vi "changeFWpos.vi"(1 "FW pos":u8, 2 "FWhandle":u32) -> (0 "fwPosChanged":bool)   [LabVIEW 2015]
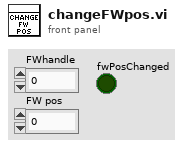
[diagram p1: front panel]
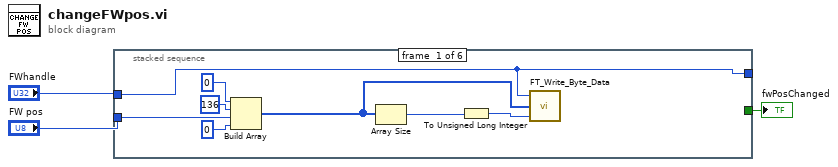
[diagram p0: block diagram]
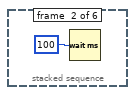
[diagram p2: hidden frame]
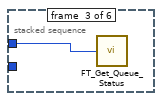
[diagram p3: hidden frame]
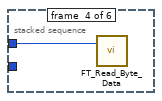
[diagram p4: hidden frame]
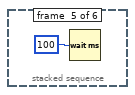
[diagram p5: hidden frame]
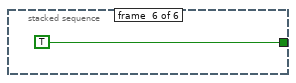
[diagram p6: hidden frame]
diagram:
  n1 = stacked-sequence {
    tunnel: "FWhandle" -> [w5 _ w13 w14 _ _]
    tunnel: [w5 _ _ _ _ _] -> _
    tunnel: "FW pos" -> [w4 _ _ _ _ _]
    tunnel: [_ _ _ _ _ TRUE] -> w1
    frame #0 {
      n2 = Build Array(u8 0 ("element"), u8 136 ("element"), w4, u8 0 ("element")) -> (w11:u8[])
      n3 = Array Size(array=w11) -> (size(s)=w9:i32)
      n4 = To Unsigned Long Integer(number=w9) -> (unsigned 32bit integer=w10:u32)
      n5 = call "FT_Write_Byte_Data.vi"("Bytes To Write"=w10, "Buffer"=w11, "Handle"=w5) -> ()  [unwired: 2 out]
    }
    frame #1 {
      n6 = Wait (ms)(milliseconds to wait=u32 100) -> ()  [unwired: 1 out]
    }
    frame #2 {
      n7 = call "FT_Get_Queue_Status.vi"("Handle"=w13) -> ()  [unwired: 2 out]
    }
    frame #3 {
      n8 = call "FT_Read_Byte_Data.vi"("Handle"=w14) -> ()  [unwired: 1 in, 3 out]
    }
    frame #4 {
      n9 = Wait (ms)(milliseconds to wait=u32 100) -> ()  [unwired: 1 out]
    }
    frame #5 {
    }
  }
  "fwPosChanged" <- w1
